vi "create_caxis_calculation_grid.vi"(8 "Error In":errorcluster) -> (0 "Error Out":errorcluster, 2 "phic":dbl[](array[numeric]), 3 "thetac":dbl[](array[numeric]))   [LabVIEW 2019]
doc: "Create a grid calculation of -90<theta c<=90 and -90<phic<=90"
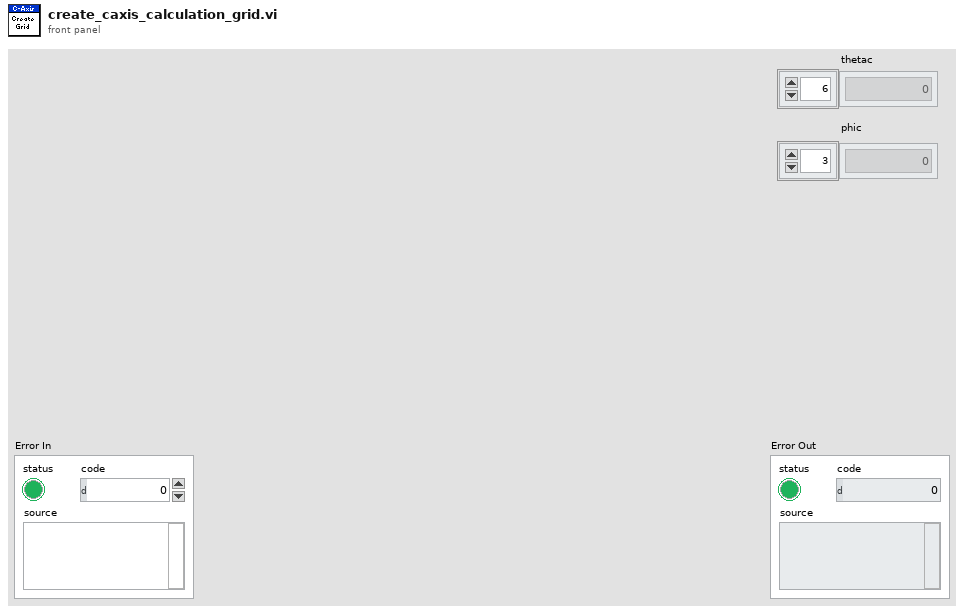
[diagram p1: front panel]
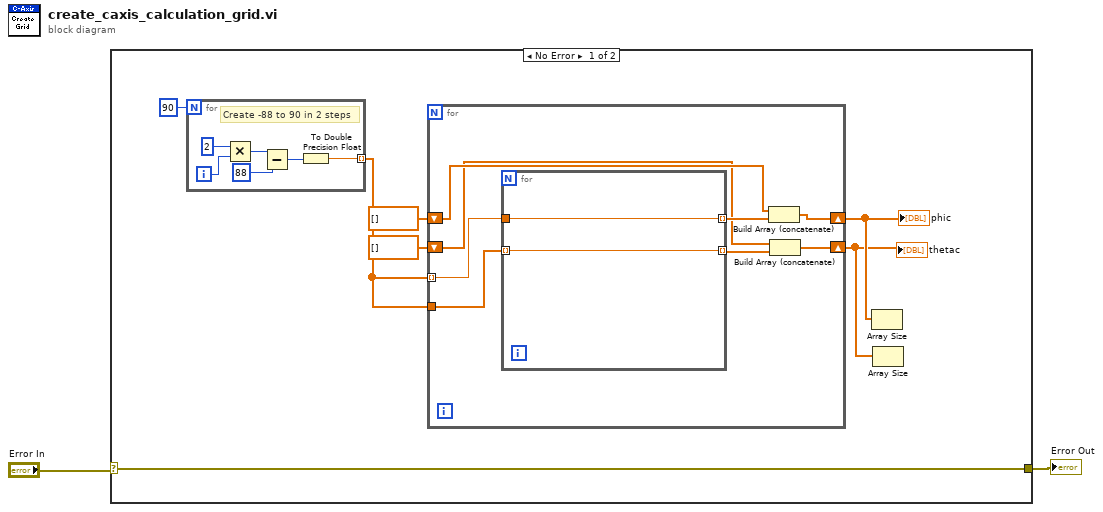
[diagram p0: block diagram]
diagram:
  n1 = case shown="No Error" "Error In" {
    selector: "Error In" -> [w9 w26]
    tunnel: [w9 w26] -> w1
    frame No Error {
      n2 = for {
        N: 90 -> [_]
        tunnel: [w20] -> w7 mode=indexing
        i -> [w25]
        # "Create -88 to 90 in 2 steps"
        n3 = Multiply(x=2, y=w25) -> (x*y=w23:i32)
        n4 = Subtract(x=w23, y=88) -> (x-y=w21:i32)
        n5 = To Double Precision Float(number=w21) -> (double precision float=w20:dbl)
      }
      n6 = for {
        tunnel: w7 -> [w17] mode=indexing
        tunnel: w7 -> [w16]
        shift-right: [w13] -> w6
        shift-left: dbl[] [] -> [w11]
        shift-right: [w12] -> w5
        shift-left: dbl[] [] -> [w10]
        n7 = for {
          tunnel: w17 -> [w19]
          tunnel: [w19] -> w14 mode=indexing
          tunnel: w16 -> [w18] mode=indexing
          tunnel: [w18] -> w15 mode=indexing
        }
        n8 = Build Array (concatenate)(w11, w14) -> (w13:dbl[])
        n9 = Build Array (concatenate)(w10, w15) -> (w12:dbl[])
      }
      "phic" <- w6
      "thetac" <- w5
      n10 = Array Size(array=w6) -> ()  [unwired: 1 out]
      n11 = Array Size(array=w5) -> ()  [unwired: 1 out]
    }
    frame Error {
    }
  }
  "Error Out" <- w1
